vi "Lab Panel V5.20.vi"() -> ()   [LabVIEW 2013] (continued)
                                n577 = call <vilib>:"Clear Errors.vi"("error in (no error)"=w882) -> ()  [unwired: 6 in, 1 out]
                                n578 = global write "Global 1.vi" "LAB01-2 FILE"(w869) -> ()
                              }
                              frame #1 {
                                (unwired) FALSE
                                n579 = String To Path(string=w893) -> (path=w889:path)
                                n580 = TDMS Open(6:FALSE, 10:T20."create or replace" ("operation (0:open)"), 11:w889) -> (0:w888:errorcluster, 3:→"TDMS LAB01-2":refnum<k34>)  [unwired: 4 in]
                              }
                              frame #2 {
                                n581 = local read "SET LAB01-2"() -> (w899:T5)
                                n582 = local read "TDMS LAB01-2"() -> (w910:refnum<k34>)
                                n583 = Build Array("Testers Name", "Description", "Set Test Cycles", "T-Rise minutes", "T-Rise Deg C") -> (w900:string[])
                                n584 = Unbundle(w899) -> ("NAME"=w898:string, "DESCRIPTION"=w897:string, "CYCLES"=w896:dbl, "T-RISE mins"=w895:dbl, "T-RISE deg C"=w894:dbl)
                                n585 = Number To Decimal String(number=w896) -> (decimal integer string=w909:string)  [unwired: 1 in]
                                n586 = Number To Decimal String(number=w895) -> (decimal integer string=w908:string)  [unwired: 1 in]
                                n587 = Number To Decimal String(number=w894) -> (decimal integer string=w907:string)  [unwired: 1 in]
                                n588 = Build Array(w898, w897, w909, w908, w907) -> (w906:string[])
                                n589 = TDMS Set Properties(5:w906, 7:w900, 11:w910) -> ()  [unwired: 3 in, 4 out]
                              }
                              frame #3 {
                                n590 = local read "DISP LAB01-2"() -> (w912:T4)
                                n591 = Concatenate Strings("LAB01-2  ", w915) -> (w916:string)
                                n592 = Two Button Dialog(message=w916, 1:w913, 2:w914) -> (T button?=w918:bool)
                                n593 = case shown="True" w918 {
                                tunnel: w912 -> [w925 w926]
                                tunnel: [w925 w926] -> w922
                                tunnel: [w924 w927] -> w921
                                tunnel: [w923 w927] -> w920
                                frame False {
                                n594 = Unbundle(w925) -> ("CYCLE"=w924:dbl, "MINS"=w923:dbl)  [unwired: 1 out]
                                }
                                frame True {
                                w927 = 0.0
                                }
                                }
                                n595 = Bundle(cluster=w922, "CYCLE"=w921, "MINS"=w920, "STATUS"="RUN") -> (w911:T4)
                                n596 = local write "DISP LAB01-2"(w911) -> ()
                              }
                              frame #4 {
                                n597 = local read "TEMP START LAB01-2"() -> (w930:cluster{"TL":dbl, "TN":dbl})
                                n598 = Bundle(cluster=w930, "TL"=w928, "TN"=w928) -> (w929:cluster{"TL":dbl, "TN":dbl})
                                n599 = local write "TEMP START LAB01-2"(w929) -> ()
                              }
                            }
                          }
                        }
                      }
                    }
                  }
                }
              }
              event "RUN LAB02-1": Value Change {
                n600 = event-data() -> ("NewVal"=w936:bool)  [unwired: 1 in, 5 out]
                n601 = local read "SIG LAB02-1"() -> (w932:T2)
                n602 = case shown="True" w936 {
                  tunnel: w942 -> [_ w980]
                  tunnel: w941 -> [_ w979]
                  tunnel: w939 -> [w944 w978]
                  tunnel: w940 -> [_ w977]
                  tunnel: w938 -> [_ w976]
                  tunnel: [w943 w975] -> w937
                  tunnel: w935 -> [_ w974]
                  tunnel: w934 -> [_ w973]
                  tunnel: w933 -> [_ w972]
                  tunnel: w932 -> [_ w971]
                  tunnel: w931 -> [_ w970]
                  frame False {
                    # "stop test"
                    n603 = stacked-sequence {
                      tunnel: w944 -> [w953 _]
                      tunnel: [w945 _] -> w943
                      frame #0 {
                        n604 = local read "DISP LAB02-1"() -> (w952:T4)
                        n605 = Unbundle(w952) -> ("CYCLE"=w950:dbl, "MINS"=w951:dbl)  [unwired: 1 out]
                        n606 = case shown="\"CYCLE TEST\"" w953 {
                          tunnel: w951 -> [_ _ w960]
                          tunnel: w950 -> [w958 w959 _]
                          tunnel: [w958 w959 w960] -> w949
                          frame "CHART TEST", Default {
                          }
                          frame "CYCLE TEST" {
                          }
                          frame "T-RISE TEST" {
                          }
                        }
                        n607 = local read "TDMS LAB02-1"() -> (w957:refnum<k34>)
                        n608 = Build Array("STOPPED") -> (w954:string[])
                        n609 = Build Array(w949) -> (w948:dbl[])
                        n610 = TDMS Write(0:w957, 5:"TEST RESULT", 7:w954, 9:w948) -> (4:w946:refnum<k34>, 15:w947:errorcluster)  [unwired: 2 in, 2 out]
                        n611 = TDMS Close(8:w947, 11:w946) -> (0:w945:errorcluster)  [unwired: 1 out]
                      }
                      frame #1 {
                        n612 = local read "DISP LAB02-1"() -> (w964:T4)
                        n613 = stacked-sequence {
                          tunnel: "LAB02-1" -> [w966 w968]
                          frame #0 {
                            n614 = call "sub vi - defrag tdms v1.vi"("panel id"=w966) -> ("error out"=w965:errorcluster)  [unwired: 10 in]
                            n615 = local write "data file error"(w965) -> ()
                          }
                          frame #1 {
                            n616 = local write "RESULT LAB02-1"(FALSE) -> ()
                            n617 = call "Save data file (stop) v3.vi"("panel id"=w968) -> ("network file save error"=w967:errorcluster)  [unwired: 9 in, 1 out]
                            n618 = local write "data file error"(w967) -> ()
                          }
                        }
                        n619 = Bundle(cluster=w964, "STATUS"="STOP") -> (w962:T4)  [unwired: 2 in]
                        n620 = local write "DISP LAB02-1"(w962) -> ()
                      }
                    }
                  }
                  frame True {
                    n621 = stacked-sequence {
                      seq-local: [w982 _] -> [_ w986]
                      tunnel: w980 -> [_ w996]
                      tunnel: w979 -> [_ w995]
                      tunnel: w978 -> [_ w994]
                      tunnel: w977 -> [_ w993]
                      tunnel: w976 -> [_ w992]
                      tunnel: [_ w991] -> w975
                      tunnel: w974 -> [_ w990]
                      tunnel: w973 -> [_ w989]
                      tunnel: w972 -> [_ w988]
                      tunnel: w971 -> [w981 w987]
                      tunnel: w970 -> [_ w985]
                      frame #0 {
                        n622 = Unbundle(w981) -> ("AMPS"=w984:dbl)  [unwired: 4 out]
                        n623 = call "Check For Amps on v1.vi"("ID"="LAB02-1", "amps"=w984) -> ("amps"=w982:bool)  [unwired: 9 in]
                      }
                      frame #1 {
                        n624 = case shown="True" w986 {
                          tunnel: w996 -> [_ w1009]
                          tunnel: w995 -> [_ w1008]
                          tunnel: w994 -> [_ w1007]
                          tunnel: w993 -> [_ w1006]
                          tunnel: w992 -> [_ w1005]
                          tunnel: [errorcluster {"status"=FALSE, "code"=0, "source"=""} ("error out") w1004] -> w991
                          tunnel: w990 -> [_ w1003]
                          tunnel: w989 -> [_ w1002]
                          tunnel: w988 -> [_ w1001]
                          tunnel: w987 -> [_ w1000]
                          tunnel: w985 -> [_ w999]
                          frame False {
                            w998 = FALSE
                            n625 = local write "RUN LAB02-1"(w998) -> ()
                            n626 = local write "run lab02-1"(w998) -> ()
                          }
                          frame True {
                            n627 = stacked-sequence {
                              seq-local: [w1010 _ _ _ _] -> [_ w1034 _ _ _]
                              tunnel: w1009 -> [w1015 _ _ _ _]
                              tunnel: w1008 -> [w1012 _ _ _ _]
                              tunnel: w1007 -> [w1025 _ _ _ _]
                              tunnel: w1006 -> [w1018 _ _ _ _]
                              tunnel: w1005 -> [w1013 _ _ _ _]
                              tunnel: [_ w1029 _ _ _] -> w1004
                              tunnel: w1003 -> [_ _ _ w1055 _]
                              tunnel: w1002 -> [_ _ _ w1054 _]
                              tunnel: w1001 -> [_ _ _ w1053 _]
                              tunnel: w1000 -> [_ _ _ _ _]
                              tunnel: w999 -> [_ _ _ _ w1069]
                              frame #0 {
                                w1011 = "\\"
                                n628 = local read "SET LAB02-1"() -> (w1020:T5)
                                n629 = case shown="\"CYCLE TEST\"" w1025 {
                                tunnel: ["L02-1-CHART TEST-" "L02-1-CYCLE TEST-" "L02-1-T-RISE TEST-"] -> w1021
                                frame "CHART TEST", Default {
                                }
                                frame "CYCLE TEST" {
                                }
                                frame "T-RISE TEST" {
                                }
                                }
                                n630 = Unbundle(w1020) -> ("DESCRIPTION"=w1019:string)  [unwired: 4 out]
                                n631 = Concatenate Strings(w1015, "\\", w1013, w1011, w1012, w1011) -> (w1022:string)
                                n632 = String To Path(string=w1022) -> (path=w1024:path)
                                n633 = Concatenate Strings(w1022, w1021, w1019, "-", w1018, ".tdms") -> (w1010:string)
                                n634 = Create Folder(path (use dialog)=w1024) -> (error out=w1023:errorcluster)  [unwired: 2 in, 2 out]
                                n635 = global write "Global 1.vi" "LAB02-1 FILE"(w1010) -> ()
                                n636 = call <vilib>:"Clear Errors.vi"("error in (no error)"=w1023) -> ()  [unwired: 6 in, 1 out]
                              }
                              frame #1 {
                                (unwired) FALSE
                                n637 = String To Path(string=w1034) -> (path=w1030:path)
                                n638 = TDMS Open(6:FALSE, 10:T20."create or replace" ("operation (0:open)"), 11:w1030) -> (0:w1029:errorcluster, 3:→"TDMS LAB02-1":refnum<k34>)  [unwired: 4 in]
                              }
                              frame #2 {
                                n639 = local read "SET LAB02-1"() -> (w1040:T5)
                                n640 = local read "TDMS LAB02-1"() -> (w1051:refnum<k34>)
                                n641 = Build Array("Testers Name", "Description", "Set Test Cycles", "T-Rise minutes", "T-Rise Deg C") -> (w1041:string[])
                                n642 = Unbundle(w1040) -> ("NAME"=w1039:string, "DESCRIPTION"=w1038:string, "CYCLES"=w1037:dbl, "T-RISE mins"=w1036:dbl, "T-RISE deg C"=w1035:dbl)
                                n643 = Number To Decimal String(number=w1037) -> (decimal integer string=w1050:string)  [unwired: 1 in]
                                n644 = Number To Decimal String(number=w1036) -> (decimal integer string=w1049:string)  [unwired: 1 in]
                                n645 = Number To Decimal String(number=w1035) -> (decimal integer string=w1048:string)  [unwired: 1 in]
                                n646 = Build Array(w1039, w1038, w1050, w1049, w1048) -> (w1047:string[])
                                n647 = TDMS Set Properties(5:w1047, 7:w1041, 11:w1051) -> ()  [unwired: 3 in, 4 out]
                              }
                              frame #3 {
                                n648 = local read "DISP LAB02-1"() -> (w1056:T4)
                                n649 = Concatenate Strings("LAB02-1  ", w1055) -> (w1057:string)
                                n650 = Two Button Dialog(message=w1057, 1:w1053, 2:w1054) -> (T button?=w1059:bool)
                                n651 = case shown="True" w1059 {
                                tunnel: w1056 -> [w1066 w1067]
                                tunnel: [w1066 w1067] -> w1063
                                tunnel: [w1065 w1068] -> w1062
                                tunnel: [w1064 w1068] -> w1061
                                frame False {
                                n652 = Unbundle(w1066) -> ("CYCLE"=w1065:dbl, "MINS"=w1064:dbl)  [unwired: 1 out]
                                }
                                frame True {
                                w1068 = 0.0
                                }
                                }
                                n653 = Bundle(cluster=w1063, "CYCLE"=w1062, "MINS"=w1061, "STATUS"="RUN") -> (w1052:T4)
                                n654 = local write "DISP LAB02-1"(w1052) -> ()
                              }
                              frame #4 {
                                n655 = local read "TEMP START LAB02-1"() -> (w1071:cluster{"TL":dbl, "TN":dbl})
                                n656 = Bundle(cluster=w1071, "TL"=w1069, "TN"=w1069) -> (w1070:cluster{"TL":dbl, "TN":dbl})
                                n657 = local write "TEMP START LAB02-1"(w1070) -> ()
                              }
                            }
                          }
                        }
                      }
                    }
                  }
                }
                n658 = local write "run lab02-1"(w936) -> ()
              }
              event "RUN LAB02-2": Value Change {
                n659 = event-data() -> ("NewVal"=w1076:bool)  [unwired: 1 in, 5 out]
                n660 = local write "run lab02-2"(w1076) -> ()
                n661 = case shown="True" w1076 {
                  tunnel: w1082 -> [_ w1120]
                  tunnel: w1081 -> [_ w1119]
                  tunnel: w1079 -> [w1084 w1118]
                  tunnel: w1080 -> [_ w1117]
                  tunnel: w1078 -> [_ w1116]
                  tunnel: [w1083 w1115] -> w1077
                  tunnel: w1075 -> [_ w1114]
                  tunnel: w1074 -> [_ w1113]
                  tunnel: w1073 -> [_ w1112]
                  tunnel: w1072 -> [_ w1110]
                  frame False {
                    # "stop test"
                    n662 = stacked-sequence {
                      tunnel: w1084 -> [w1093 _]
                      tunnel: [w1085 _] -> w1083
                      frame #0 {
                        n663 = local read "DISP LAB02-2"() -> (w1092:T4)
                        n664 = Unbundle(w1092) -> ("CYCLE"=w1090:dbl, "MINS"=w1091:dbl)  [unwired: 1 out]
                        n665 = case shown="\"CYCLE TEST\"" w1093 {
                          tunnel: w1091 -> [_ _ w1100]
                          tunnel: w1090 -> [w1098 w1099 _]
                          tunnel: [w1098 w1099 w1100] -> w1089
                          frame "CHART TEST", Default {
                          }
                          frame "CYCLE TEST" {
                          }
                          frame "T-RISE TEST" {
                          }
                        }
                        n666 = local read "TDMS LAB02-2"() -> (w1097:refnum<k34>)
                        n667 = Build Array("STOPPED") -> (w1094:string[])
                        n668 = Build Array(w1089) -> (w1088:dbl[])
                        n669 = TDMS Write(0:w1097, 5:"TEST RESULT", 7:w1094, 9:w1088) -> (4:w1086:refnum<k34>, 15:w1087:errorcluster)  [unwired: 2 in, 2 out]
                        n670 = TDMS Close(8:w1087, 11:w1086) -> (0:w1085:errorcluster)  [unwired: 1 out]
                      }
                      frame #1 {
                        n671 = local read "DISP LAB02-2"() -> (w1104:T4)
                        n672 = stacked-sequence {
                          tunnel: "LAB02-2" -> [w1106 w1108]
                          frame #0 {
                            n673 = call "sub vi - defrag tdms v1.vi"("panel id"=w1106) -> ("error out"=w1105:errorcluster)  [unwired: 10 in]
                            n674 = local write "data file error"(w1105) -> ()
                          }
                          frame #1 {
                            n675 = call "Save data file (stop) v3.vi"("panel id"=w1108) -> ("network file save error"=w1107:errorcluster)  [unwired: 9 in, 1 out]
                            n676 = local write "RESULT LAB02-2"(FALSE) -> ()
                            n677 = local write "data file error"(w1107) -> ()
                          }
                        }
                        n678 = Bundle(cluster=w1104, "STATUS"="STOP") -> (w1102:T4)  [unwired: 2 in]
                        n679 = local write "DISP LAB02-2"(w1102) -> ()
                      }
                    }
                  }
                  frame True {
                    n680 = local read "SIG LAB02-2"() -> (w1111:T2)
                    n681 = stacked-sequence {
                      seq-local: [w1122 _] -> [_ w1126]
                      tunnel: w1120 -> [_ w1136]
                      tunnel: w1119 -> [_ w1135]
                      tunnel: w1118 -> [_ w1134]
                      tunnel: w1117 -> [_ w1133]
                      tunnel: w1116 -> [_ w1132]
                      tunnel: [_ w1131] -> w1115
                      tunnel: w1114 -> [_ w1130]
                      tunnel: w1113 -> [_ w1129]
                      tunnel: w1112 -> [_ w1128]
                      tunnel: w1111 -> [w1121 w1127]
                      tunnel: w1110 -> [_ w1125]
                      frame #0 {
                        n682 = Unbundle(w1121) -> ("AMPS"=w1124:dbl)  [unwired: 4 out]
                        n683 = call "Check For Amps on v1.vi"("ID"="LAB02-2", "amps"=w1124) -> ("amps"=w1122:bool)  [unwired: 9 in]
                      }
                      frame #1 {
                        n684 = case shown="True" w1126 {
                          tunnel: w1136 -> [_ w1149]
                          tunnel: w1135 -> [_ w1148]
                          tunnel: w1134 -> [_ w1147]
                          tunnel: w1133 -> [_ w1146]
                          tunnel: w1132 -> [_ w1145]
                          tunnel: [errorcluster {"status"=FALSE, "code"=0, "source"=""} ("error out") w1144] -> w1131
                          tunnel: w1130 -> [_ w1143]
                          tunnel: w1129 -> [_ w1142]
                          tunnel: w1128 -> [_ w1141]
                          tunnel: w1127 -> [_ w1140]
                          tunnel: w1125 -> [_ w1139]
                          frame False {
                            w1137 = FALSE
                            n685 = local write "RUN LAB02-2"(w1137) -> ()
                            n686 = local write "run lab02-2"(w1137) -> ()
                          }
                          frame True {
                            n687 = stacked-sequence {
                              seq-local: [w1150 _ _ _ _] -> [_ w1174 _ _ _]
                              tunnel: w1149 -> [w1155 _ _ _ _]
                              tunnel: w1148 -> [w1152 _ _ _ _]
                              tunnel: w1147 -> [w1165 _ _ _ _]
                              tunnel: w1146 -> [w1158 _ _ _ _]
                              tunnel: w1145 -> [w1153 _ _ _ _]
                              tunnel: [_ w1169 _ _ _] -> w1144
                              tunnel: w1143 -> [_ _ _ w1195 _]
                              tunnel: w1142 -> [_ _ _ w1194 _]
                              tunnel: w1141 -> [_ _ _ w1193 _]
                              tunnel: w1140 -> [_ _ _ _ _]
                              tunnel: w1139 -> [_ _ _ _ w1209]
                              frame #0 {
                                w1151 = "\\"
                                n688 = local read "SET LAB02-2"() -> (w1160:T5)
                                n689 = case shown="\"CYCLE TEST\"" w1165 {
                                tunnel: ["L02-2-CHART TEST-" "L02-2-CYCLE TEST-" "L02-2-T-RISE TEST-"] -> w1161
                                frame "CHART TEST", Default {
                                }
                                frame "CYCLE TEST" {
                                }
                                frame "T-RISE TEST" {
                                }
                                }
                                n690 = Unbundle(w1160) -> ("DESCRIPTION"=w1159:string)  [unwired: 4 out]
                                n691 = Concatenate Strings(w1155, "\\", w1153, w1151, w1152, w1151) -> (w1162:string)
                                n692 = String To Path(string=w1162) -> (path=w1164:path)
                                n693 = Concatenate Strings(w1162, w1161, w1159, "-", w1158, ".tdms") -> (w1150:string)
                                n694 = Create Folder(path (use dialog)=w1164) -> (error out=w1163:errorcluster)  [unwired: 2 in, 2 out]
                                n695 = global write "Global 1.vi" "LAB02-2 FILE"(w1150) -> ()
                                n696 = call <vilib>:"Clear Errors.vi"("error in (no error)"=w1163) -> ()  [unwired: 6 in, 1 out]
                              }
                              frame #1 {
                                (unwired) FALSE
                                n697 = String To Path(string=w1174) -> (path=w1170:path)
                                n698 = TDMS Open(6:FALSE, 10:T20."create or replace" ("operation (0:open)"), 11:w1170) -> (0:w1169:errorcluster, 3:→"TDMS LAB02-2":refnum<k34>)  [unwired: 4 in]
                              }
                              frame #2 {
                                n699 = local read "SET LAB02-2"() -> (w1180:T5)
                                n700 = local read "TDMS LAB02-2"() -> (w1191:refnum<k34>)
                                n701 = Build Array("Testers Name", "Description", "Set Test Cycles", "T-Rise minutes", "T-Rise Deg C") -> (w1181:string[])
                                n702 = Unbundle(w1180) -> ("NAME"=w1179:string, "DESCRIPTION"=w1178:string, "CYCLES"=w1177:dbl, "T-RISE mins"=w1176:dbl, "T-RISE deg C"=w1175:dbl)
                                n703 = Number To Decimal String(number=w1177) -> (decimal integer string=w1190:string)  [unwired: 1 in]
                                n704 = Number To Decimal String(number=w1176) -> (decimal integer string=w1189:string)  [unwired: 1 in]
                                n705 = Number To Decimal String(number=w1175) -> (decimal integer string=w1188:string)  [unwired: 1 in]
                                n706 = Build Array(w1179, w1178, w1190, w1189, w1188) -> (w1187:string[])
                                n707 = TDMS Set Properties(5:w1187, 7:w1181, 11:w1191) -> ()  [unwired: 3 in, 4 out]
                              }
                              frame #3 {
                                n708 = local read "DISP LAB02-2"() -> (w1196:T4)
                                n709 = Concatenate Strings("LAB02-2  ", w1195) -> (w1197:string)
                                n710 = Two Button Dialog(message=w1197, 1:w1193, 2:w1194) -> (T button?=w1199:bool)
                                n711 = case shown="True" w1199 {
                                tunnel: w1196 -> [w1206 w1207]
                                tunnel: [w1206 w1207] -> w1203
                                tunnel: [w1205 w1208] -> w1202
                                tunnel: [w1204 w1208] -> w1201
                                frame False {
                                n712 = Unbundle(w1206) -> ("CYCLE"=w1205:dbl, "MINS"=w1204:dbl)  [unwired: 1 out]
                                }
                                frame True {
                                w1208 = 0.0
                                }
                                }
                                n713 = Bundle(cluster=w1203, "CYCLE"=w1202, "MINS"=w1201, "STATUS"="RUN") -> (w1192:T4)
                                n714 = local write "DISP LAB02-2"(w1192) -> ()
                              }
                              frame #4 {
                                n715 = local read "TEMP START LAB02-2"() -> (w1211:cluster{"TL":dbl, "TN":dbl})
                                n716 = Bundle(cluster=w1211, "TL"=w1209, "TN"=w1209) -> (w1210:cluster{"TL":dbl, "TN":dbl})
                                n717 = local write "TEMP START LAB02-2"(w1210) -> ()
                              }
                            }
                          }
                        }
                      }
                    }
                  }
                }
              }
              event "RUN LAB03-1": Value Change {
                n718 = event-data() -> ("NewVal"=w1216:bool)  [unwired: 1 in, 5 out]
                n719 = local write "run lab03-1"(w1216) -> ()
                n720 = case shown="True" w1216 {
                  tunnel: w1222 -> [_ w1260]
                  tunnel: w1221 -> [_ w1259]
                  tunnel: w1219 -> [w1224 w1258]
                  tunnel: w1220 -> [_ w1257]
                  tunnel: w1218 -> [_ w1256]
                  tunnel: [w1223 w1255] -> w1217
                  tunnel: w1215 -> [_ w1254]
                  tunnel: w1214 -> [_ w1253]
                  tunnel: w1213 -> [_ w1252]
                  tunnel: w1212 -> [_ w1250]
                  frame False {
                    # "stop test"
                    n721 = stacked-sequence {
                      tunnel: w1224 -> [w1233 _]
                      tunnel: [w1225 _] -> w1223
                      frame #0 {
                        n722 = local read "DISP LAB03-1"() -> (w1232:T4)
                        n723 = Unbundle(w1232) -> ("CYCLE"=w1230:dbl, "MINS"=w1231:dbl)  [unwired: 1 out]
                        n724 = case shown="\"CYCLE TEST\"" w1233 {
                          tunnel: w1231 -> [_ _ w1240]
                          tunnel: w1230 -> [w1238 w1239 _]
                          tunnel: [w1238 w1239 w1240] -> w1229
                          frame "CHART TEST", Default {
                          }
                          frame "CYCLE TEST" {
                          }
                          frame "T-RISE TEST" {
                          }
                        }
                        n725 = local read "TDMS LAB03-1"() -> (w1237:refnum<k34>)
                        n726 = Build Array("STOPPED") -> (w1234:string[])
                        n727 = Build Array(w1229) -> (w1228:dbl[])
                        n728 = TDMS Write(0:w1237, 5:"TEST RESULT", 7:w1234, 9:w1228) -> (4:w1226:refnum<k34>, 15:w1227:errorcluster)  [unwired: 2 in, 2 out]
                        n729 = TDMS Close(8:w1227, 11:w1226) -> (0:w1225:errorcluster)  [unwired: 1 out]
                      }
                      frame #1 {
                        n730 = local read "DISP LAB03-1"() -> (w1244:T4)
                        n731 = stacked-sequence {
                          tunnel: "LAB03-1" -> [w1246 w1248]
                          frame #0 {
                            n732 = call "sub vi - defrag tdms v1.vi"("panel id"=w1246) -> ("error out"=w1245:errorcluster)  [unwired: 10 in]
                            n733 = local write "data file error"(w1245) -> ()
                          }
                          frame #1 {
                            n734 = call "Save data file (stop) v3.vi"("panel id"=w1248) -> ("network file save error"=w1247:errorcluster)  [unwired: 9 in, 1 out]
                            n735 = local write "RESULT LAB03-1"(FALSE) -> ()
                            n736 = local write "data file error"(w1247) -> ()
                          }
                        }
                        n737 = Bundle(cluster=w1244, "STATUS"="STOP") -> (w1242:T4)  [unwired: 2 in]
                        n738 = local write "DISP LAB03-1"(w1242) -> ()
                      }
                    }
                  }
                  frame True {
                    n739 = local read "SIG LAB03-1"() -> (w1251:T2)
                    n740 = stacked-sequence {
                      seq-local: [w1262 _] -> [_ w1266]
                      tunnel: w1260 -> [_ w1276]
                      tunnel: w1259 -> [_ w1275]
                      tunnel: w1258 -> [_ w1274]
                      tunnel: w1257 -> [_ w1273]
                      tunnel: w1256 -> [_ w1272]
                      tunnel: [_ w1271] -> w1255
                      tunnel: w1254 -> [_ w1270]
                      tunnel: w1253 -> [_ w1269]
                      tunnel: w1252 -> [_ w1268]
                      tunnel: w1251 -> [w1261 w1267]
                      tunnel: w1250 -> [_ w1265]
                      frame #0 {
                        n741 = Unbundle(w1261) -> ("AMPS"=w1264:dbl)  [unwired: 4 out]
                        n742 = call "Check For Amps on v1.vi"("ID"="LAB03-1", "amps"=w1264) -> ("amps"=w1262:bool)  [unwired: 9 in]
                      }
                      frame #1 {
                        n743 = case shown="True" w1266 {
                          tunnel: w1276 -> [_ w1289]
                          tunnel: w1275 -> [_ w1288]
                          tunnel: w1274 -> [_ w1287]
                          tunnel: w1273 -> [_ w1286]
                          tunnel: w1272 -> [_ w1285]
                          tunnel: [errorcluster {"status"=FALSE, "code"=0, "source"=""} ("error out") w1284] -> w1271
                          tunnel: w1270 -> [_ w1283]
                          tunnel: w1269 -> [_ w1282]
                          tunnel: w1268 -> [_ w1281]
                          tunnel: w1267 -> [_ w1280]
                          tunnel: w1265 -> [_ w1279]
                          frame False {
                            w1277 = FALSE
                            n744 = local write "RUN LAB03-1"(w1277) -> ()
                            n745 = local write "run lab03-1"(w1277) -> ()
                          }
                          frame True {
                            n746 = stacked-sequence {
                              seq-local: [w1290 _ _ _ _] -> [_ w1314 _ _ _]
                              tunnel: w1289 -> [w1295 _ _ _ _]
                              tunnel: w1288 -> [w1292 _ _ _ _]
                              tunnel: w1287 -> [w1305 _ _ _ _]
                              tunnel: w1286 -> [w1298 _ _ _ _]
                              tunnel: w1285 -> [w1293 _ _ _ _]
                              tunnel: [_ w1309 _ _ _] -> w1284
                              tunnel: w1283 -> [_ _ _ w1334 _]
                              tunnel: w1282 -> [_ _ _ w1333 _]
                              tunnel: w1281 -> [_ _ _ w1332 _]
                              tunnel: w1280 -> [_ _ _ _ _]
                              tunnel: w1279 -> [_ _ _ _ w1349]
                              frame #0 {
                                w1291 = "\\"
                                n747 = local read "SET LAB03-1"() -> (w1300:T5)
                                n748 = case shown="\"T-RISE TEST\"" w1305 {
                                tunnel: ["L03-1-CHART TEST-" "L03-1-CYCLE TEST-" "L03-1-T-RISE TEST-"] -> w1301
                                frame "CHART TEST", Default {
                                }
                                frame "CYCLE TEST" {
                                }
                                frame "T-RISE TEST" {
                                }
                                }
                                n749 = Unbundle(w1300) -> ("DESCRIPTION"=w1299:string)  [unwired: 4 out]
                                n750 = Concatenate Strings(w1295, "\\", w1293, w1291, w1292, w1291) -> (w1302:string)
                                n751 = String To Path(string=w1302) -> (path=w1304:path)
                                n752 = Concatenate Strings(w1302, w1301, w1299, "-", w1298, ".tdms") -> (w1290:string)
                                n753 = Create Folder(path (use dialog)=w1304) -> (error out=w1303:errorcluster)  [unwired: 2 in, 2 out]
                                n754 = global write "Global 1.vi" "LAB03-1 FILE"(w1290) -> ()
                                n755 = call <vilib>:"Clear Errors.vi"("error in (no error)"=w1303) -> ()  [unwired: 6 in, 1 out]
                              }
                              frame #1 {
                                (unwired) FALSE
                                n756 = String To Path(string=w1314) -> (path=w1310:path)
                                n757 = TDMS Open(6:FALSE, 10:T20."create or replace" ("operation (0:open)"), 11:w1310) -> (0:w1309:errorcluster, 3:→"TDMS LAB03-1":refnum<k34>)  [unwired: 4 in]
                              }
                              frame #2 {
                                n758 = local read "SET LAB03-1"() -> (w1320:T5)
                                n759 = local read "TDMS LAB03-1"() -> (w1331:refnum<k34>)
                                n760 = Build Array("Testers Name", "Description", "Set Test Cycles", "T-Rise minutes", "T-Rise Deg C") -> (w1321:string[])
                                n761 = Unbundle(w1320) -> ("NAME"=w1319:string, "DESCRIPTION"=w1318:string, "CYCLES"=w1317:dbl, "T-RISE mins"=w1316:dbl, "T-RISE deg C"=w1315:dbl)
                                n762 = Number To Decimal String(number=w1317) -> (decimal integer string=w1330:string)  [unwired: 1 in]
                                n763 = Number To Decimal String(number=w1316) -> (decimal integer string=w1329:string)  [unwired: 1 in]
                                n764 = Number To Decimal String(number=w1315) -> (decimal integer string=w1328:string)  [unwired: 1 in]
                                n765 = Build Array(w1319, w1318, w1330, w1329, w1328) -> (w1327:string[])
                                n766 = TDMS Set Properties(5:w1327, 7:w1321, 11:w1331) -> ()  [unwired: 3 in, 4 out]
                              }
                              frame #3 {
                                n767 = local read "DISP LAB03-1"() -> (w1336:T4)
                                n768 = Concatenate Strings("LAB03-1  ", w1334) -> (w1337:string)
                                n769 = Two Button Dialog(message=w1337, 1:w1332, 2:w1333) -> (T button?=w1339:bool)
                                n770 = case shown="True" w1339 {
                                tunnel: w1336 -> [w1346 w1347]
                                tunnel: [w1346 w1347] -> w1343
                                tunnel: [w1345 w1348] -> w1342
                                tunnel: [w1344 w1348] -> w1341
                                frame False {
                                n771 = Unbundle(w1346) -> ("CYCLE"=w1345:dbl, "MINS"=w1344:dbl)  [unwired: 1 out]
                                }
                                frame True {
                                w1348 = 0.0
                                }
                                }
                                n772 = Bundle(cluster=w1343, "CYCLE"=w1342, "MINS"=w1341, "STATUS"="RUN") -> (w1335:T4)
                                n773 = local write "DISP LAB03-1"(w1335) -> ()
                              }
                              frame #4 {
                                n774 = local read "TEMP START LAB03-1"() -> (w1351:cluster{"TL":dbl, "TN":dbl})
                                n775 = Bundle(cluster=w1351, "TL"=w1349, "TN"=w1349) -> (w1350:cluster{"TL":dbl, "TN":dbl})
                                n776 = local write "TEMP START LAB03-1"(w1350) -> ()
                              }
                            }
                          }
                        }
                      }
                    }
                  }
                }
              }
              event "RUN LAB03-2": Value Change {
                n777 = event-data() -> ("NewVal"=w1356:bool)  [unwired: 1 in, 5 out]
                n778 = local write "run lab03-2"(w1356) -> ()
                n779 = case shown="True" w1356 {
                  tunnel: w1362 -> [_ w1400]
                  tunnel: w1361 -> [_ w1399]
                  tunnel: w1359 -> [w1364 w1398]
                  tunnel: w1360 -> [_ w1397]
                  tunnel: w1358 -> [_ w1396]
                  tunnel: [w1363 w1395] -> w1357
                  tunnel: w1355 -> [_ w1394]
                  tunnel: w1354 -> [_ w1393]
                  tunnel: w1353 -> [_ w1392]
                  tunnel: w1352 -> [_ w1390]
                  frame False {
                    # "stop test"
                    n780 = stacked-sequence {
                      tunnel: w1364 -> [w1373 _]
                      tunnel: [w1365 _] -> w1363
                      frame #0 {
                        n781 = local read "DISP LAB03-2"() -> (w1372:T4)
                        n782 = Unbundle(w1372) -> ("CYCLE"=w1370:dbl, "MINS"=w1371:dbl)  [unwired: 1 out]
                        n783 = case shown="\"CYCLE TEST\"" w1373 {
                          tunnel: w1371 -> [_ _ w1380]
                          tunnel: w1370 -> [w1378 w1379 _]
                          tunnel: [w1378 w1379 w1380] -> w1369
                          frame "CHART TEST", Default {
                          }
                          frame "CYCLE TEST" {
                          }
                          frame "T-RISE TEST" {
                          }
                        }
                        n784 = local read "TDMS LAB03-2"() -> (w1377:refnum<k34>)
                        n785 = Build Array("STOPPED") -> (w1374:string[])
                        n786 = Build Array(w1369) -> (w1368:dbl[])
                        n787 = TDMS Write(0:w1377, 5:"TEST RESULT", 7:w1374, 9:w1368) -> (4:w1366:refnum<k34>, 15:w1367:errorcluster)  [unwired: 2 in, 2 out]
                        n788 = TDMS Close(8:w1367, 11:w1366) -> (0:w1365:errorcluster)  [unwired: 1 out]
                      }
                      frame #1 {
                        n789 = local read "DISP LAB03-2"() -> (w1384:T4)
                        n790 = stacked-sequence {
                          tunnel: "LAB03-2" -> [w1386 w1388]
                          frame #0 {
                            n791 = call "sub vi - defrag tdms v1.vi"("panel id"=w1386) -> ("error out"=w1385:errorcluster)  [unwired: 10 in]
                            n792 = local write "data file error"(w1385) -> ()
                          }
                          frame #1 {
                            n793 = call "Save data file (stop) v3.vi"("panel id"=w1388) -> ("network file save error"=w1387:errorcluster)  [unwired: 9 in, 1 out]
                            n794 = local write "RESULT LAB03-2"(FALSE) -> ()
                            n795 = local write "data file error"(w1387) -> ()
                          }
                        }
                        n796 = Bundle(cluster=w1384, "STATUS"="STOP") -> (w1382:T4)  [unwired: 2 in]
                        n797 = local write "DISP LAB03-2"(w1382) -> ()
                      }
                    }
                  }
                  frame True {
                    n798 = local read "SIG LAB03-2"() -> (w1391:T2)
                    n799 = stacked-sequence {
                      seq-local: [w1402 _] -> [_ w1406]
                      tunnel: w1400 -> [_ w1416]
                      tunnel: w1399 -> [_ w1415]
                      tunnel: w1398 -> [_ w1414]
                      tunnel: w1397 -> [_ w1413]
                      tunnel: w1396 -> [_ w1412]
                      tunnel: [_ w1411] -> w1395
                      tunnel: w1394 -> [_ w1410]
                      tunnel: w1393 -> [_ w1409]
                      tunnel: w1392 -> [_ w1408]
                      tunnel: w1391 -> [w1401 w1407]
                      tunnel: w1390 -> [_ w1405]
                      frame #0 {
                        n800 = Unbundle(w1401) -> ("AMPS"=w1404:dbl)  [unwired: 4 out]
                        n801 = call "Check For Amps on v1.vi"("ID"="LAB03-2", "amps"=w1404) -> ("amps"=w1402:bool)  [unwired: 9 in]
                      }
                      frame #1 {
                        n802 = case shown="True" w1406 {
                          tunnel: w1416 -> [_ w1429]
                          tunnel: w1415 -> [_ w1428]
                          tunnel: w1414 -> [_ w1427]
                          tunnel: w1413 -> [_ w1426]
                          tunnel: w1412 -> [_ w1425]
                          tunnel: [errorcluster {"status"=FALSE, "code"=0, "source"=""} ("error out") w1424] -> w1411
                          tunnel: w1410 -> [_ w1423]
                          tunnel: w1409 -> [_ w1422]
                          tunnel: w1408 -> [_ w1421]
                          tunnel: w1407 -> [_ w1420]
                          tunnel: w1405 -> [_ w1419]
                          frame False {
                            w1417 = FALSE
                            n803 = local write "RUN LAB03-2"(w1417) -> ()
                            n804 = local write "run lab03-2"(w1417) -> ()
                          }
                          frame True {
                            n805 = stacked-sequence {
                              seq-local: [w1430 _ _ _ _] -> [_ w1454 _ _ _]
                              tunnel: w1429 -> [w1435 _ _ _ _]
                              tunnel: w1428 -> [w1432 _ _ _ _]
                              tunnel: w1427 -> [w1445 _ _ _ _]
                              tunnel: w1426 -> [w1438 _ _ _ _]
                              tunnel: w1425 -> [w1433 _ _ _ _]
                              tunnel: [_ w1449 _ _ _] -> w1424
                              tunnel: w1423 -> [_ _ _ w1475 _]
                              tunnel: w1422 -> [_ _ _ w1474 _]
                              tunnel: w1421 -> [_ _ _ w1473 _]
                              tunnel: w1420 -> [_ _ _ _ _]
                              tunnel: w1419 -> [_ _ _ _ w1489]
                              frame #0 {
                                w1431 = "\\"
                                n806 = local read "SET LAB03-2"() -> (w1440:T5)
                                n807 = case shown="\"T-RISE TEST\"" w1445 {
                                tunnel: ["L03-2-CHART TEST-" "L03-2-CYCLE TEST-" "L03-2-T-RISE TEST-"] -> w1441
                                frame "CHART TEST", Default {
                                }
                                frame "CYCLE TEST" {
                                }
                                frame "T-RISE TEST" {
                                }
                                }
                                n808 = Unbundle(w1440) -> ("DESCRIPTION"=w1439:string)  [unwired: 4 out]
                                n809 = Concatenate Strings(w1435, "\\", w1433, w1431, w1432, w1431) -> (w1442:string)
                                n810 = String To Path(string=w1442) -> (path=w1444:path)
                                n811 = Concatenate Strings(w1442, w1441, w1439, "-", w1438, ".tdms") -> (w1430:string)
                                n812 = Create Folder(path (use dialog)=w1444) -> (error out=w1443:errorcluster)  [unwired: 2 in, 2 out]
                                n813 = global write "Global 1.vi" "LAB03-2 FILE"(w1430) -> ()
                                n814 = call <vilib>:"Clear Errors.vi"("error in (no error)"=w1443) -> ()  [unwired: 6 in, 1 out]
                              }
                              frame #1 {
                                (unwired) FALSE
                                n815 = String To Path(string=w1454) -> (path=w1450:path)
                                n816 = TDMS Open(6:FALSE, 10:T20."create or replace" ("operation (0:open)"), 11:w1450) -> (0:w1449:errorcluster, 3:→"TDMS LAB03-2":refnum<k34>)  [unwired: 4 in]
                              }
                              frame #2 {
                                n817 = local read "SET LAB03-2"() -> (w1460:T5)
                                n818 = local read "TDMS LAB03-2"() -> (w1471:refnum<k34>)
                                n819 = Build Array("Testers Name", "Description", "Set Test Cycles", "T-Rise minutes", "T-Rise Deg C") -> (w1461:string[])
                                n820 = Unbundle(w1460) -> ("NAME"=w1459:string, "DESCRIPTION"=w1458:string, "CYCLES"=w1457:dbl, "T-RISE mins"=w1456:dbl, "T-RISE deg C"=w1455:dbl)
                                n821 = Number To Decimal String(number=w1457) -> (decimal integer string=w1470:string)  [unwired: 1 in]
                                n822 = Number To Decimal String(number=w1456) -> (decimal integer string=w1469:string)  [unwired: 1 in]
                                n823 = Number To Decimal String(number=w1455) -> (decimal integer string=w1468:string)  [unwired: 1 in]
                                n824 = Build Array(w1459, w1458, w1470, w1469, w1468) -> (w1467:string[])
                                n825 = TDMS Set Properties(5:w1467, 7:w1461, 11:w1471) -> ()  [unwired: 3 in, 4 out]
                              }
                              frame #3 {
                                n826 = local read "DISP LAB03-2"() -> (w1476:T4)
                                n827 = Concatenate Strings("LAB03-2  ", w1475) -> (w1477:string)
                                n828 = Two Button Dialog(message=w1477, 1:w1473, 2:w1474) -> (T button?=w1479:bool)
                                n829 = case shown="True" w1479 {
                                tunnel: w1476 -> [w1486 w1487]
                                tunnel: [w1486 w1487] -> w1483
                                tunnel: [w1485 w1488] -> w1482
                                tunnel: [w1484 w1488] -> w1481
                                frame False {
                                n830 = Unbundle(w1486) -> ("CYCLE"=w1485:dbl, "MINS"=w1484:dbl)  [unwired: 1 out]
                                }
                                frame True {
                                w1488 = 0.0
                                }
                                }
                                n831 = Bundle(cluster=w1483, "CYCLE"=w1482, "MINS"=w1481, "STATUS"="RUN") -> (w1472:T4)
                                n832 = local write "DISP LAB03-2"(w1472) -> ()
                              }
                              frame #4 {
                                n833 = local read "TEMP START LAB03-2"() -> (w1491:cluster{"TL":dbl, "TN":dbl})
                                n834 = Bundle(cluster=w1491, "TL"=w1489, "TN"=w1489) -> (w1490:cluster{"TL":dbl, "TN":dbl})
                                n835 = local write "TEMP START LAB03-2"(w1490) -> ()
                              }
                            }
                          }
                        }
                      }
                    }
                  }
                }
              }
              event "RUN LAB04-1": Value Change {
                n836 = event-data() -> ("NewVal"=w1496:bool)  [unwired: 1 in, 5 out]
                n837 = local write "run lab04-1"(w1496) -> ()
                n838 = case shown="True" w1496 {
                  tunnel: w1502 -> [_ w1540]
                  tunnel: w1501 -> [_ w1539]
                  tunnel: w1499 -> [w1504 w1538]
                  tunnel: w1500 -> [_ w1537]
                  tunnel: w1498 -> [_ w1536]
                  tunnel: [w1503 w1535] -> w1497
                  tunnel: w1495 -> [_ w1534]
                  tunnel: w1494 -> [_ w1533]
                  tunnel: w1493 -> [_ w1532]
                  tunnel: w1492 -> [_ w1530]
                  frame False {
                    # "stop test"
                    n839 = stacked-sequence {
                      tunnel: w1504 -> [w1513 _]
                      tunnel: [w1505 _] -> w1503
                      frame #0 {
                        n840 = local read "DISP LAB04-1"() -> (w1512:T4)
                        n841 = Unbundle(w1512) -> ("CYCLE"=w1510:dbl, "MINS"=w1511:dbl)  [unwired: 1 out]
                        n842 = case shown="\"CYCLE TEST\"" w1513 {
                          tunnel: w1511 -> [_ _ w1520]
                          tunnel: w1510 -> [w1518 w1519 _]
                          tunnel: [w1518 w1519 w1520] -> w1509
                          frame "CHART TEST", Default {
                          }
                          frame "CYCLE TEST" {
                          }
                          frame "T-RISE TEST" {
                          }
                        }
                        n843 = local read "TDMS LAB04-1"() -> (w1517:refnum<k34>)
                        n844 = Build Array("STOPPED") -> (w1514:string[])
                        n845 = Build Array(w1509) -> (w1508:dbl[])
                        n846 = TDMS Write(0:w1517, 5:"TEST RESULT", 7:w1514, 9:w1508) -> (4:w1506:refnum<k34>, 15:w1507:errorcluster)  [unwired: 2 in, 2 out]
                        n847 = TDMS Close(8:w1507, 11:w1506) -> (0:w1505:errorcluster)  [unwired: 1 out]
                      }
                      frame #1 {
                        n848 = local read "DISP LAB04-1"() -> (w1524:T4)
                        n849 = stacked-sequence {
                          tunnel: "LAB04-1" -> [w1526 w1528]
                          frame #0 {
                            n850 = call "sub vi - defrag tdms v1.vi"("panel id"=w1526) -> ("error out"=w1525:errorcluster)  [unwired: 10 in]
                            n851 = local write "data file error"(w1525) -> ()
                          }
                          frame #1 {
